vi "Write Subdiagrams.vi"(8 "error in (no error)":errorcluster, 10 "Subdiagrams":map{u64, T1}(c390), 11 "MultiDiagramStructure in":refnum<class "MultiDiagramStructure.lvclass">) -> (0 "error out":errorcluster, 3 "MultiDiagramStructure out":refnum<class "MultiDiagramStructure.lvclass">)   [LabVIEW 2025, in "MultiDiagramStructure.lvclass"]
uses:
  MultiDiagramStructure.lvclass
  Subdiagram.ctl
  MultiDiagramStructure.lvclass/MultiDiagramStructure.ctl
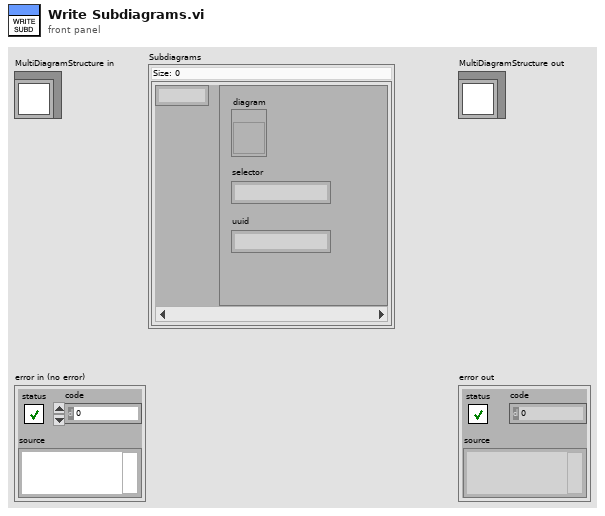
[diagram p1: front panel]
types:
  T1 = typedef "Subdiagram.ctl" = cluster{"diagram":refnum<vi>, "selector":string, "uuid":string}
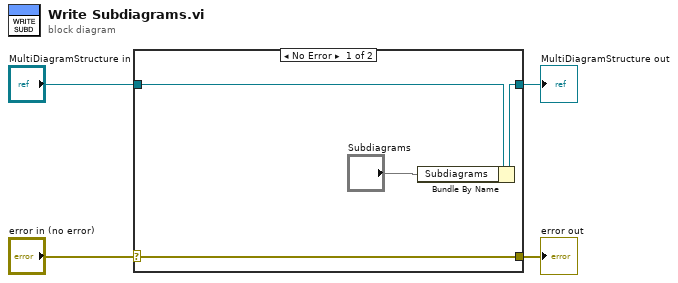
[diagram p0: block diagram]
diagram:
  n1 = case shown="No Error" "error in (no error)" {
    selector: "error in (no error)" -> [w8 w9]
    tunnel: [w8 w9] -> w3
    tunnel: [w6 w10] -> w1
    tunnel: "MultiDiagramStructure in" -> [w7 w10]
    frame No Error {
      n2 = Bundle By Name(cluster=w7, "Subdiagrams"="Subdiagrams") -> (w6:refnum<class "MultiDiagramStructure.lvclass">)
    }
    frame Error {
    }
  }
  "error out" <- w3
  "MultiDiagramStructure out" <- w1
